vi "Write Main Pane.vi"(10 "Main Pane":refnum<vi>, 11 "Flex UI in":refnum<class "Flex UI.lvclass">) -> (3 "Flex UI out":refnum<class "Flex UI.lvclass">)   [LabVIEW 2016, in "Flex UI.lvclass"]
uses:
  Flex UI.lvclass
  Flex UI.lvclass/Flex UI.ctl
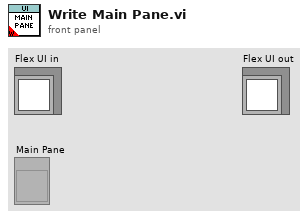
[diagram p1: front panel]
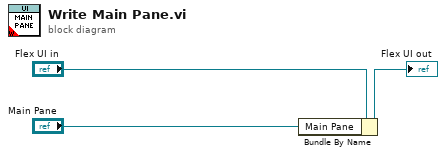
[diagram p0: block diagram]
diagram:
  n1 = Bundle By Name(cluster="Flex UI in", "Main Pane"="Main Pane") -> (→"Flex UI out":refnum<class "Flex UI.lvclass">)
